vi "Untitled 1 (SubVI).vi"(11 "input string":string) -> ()   [LabVIEW 2017]
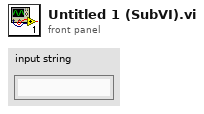
[diagram p1: front panel]
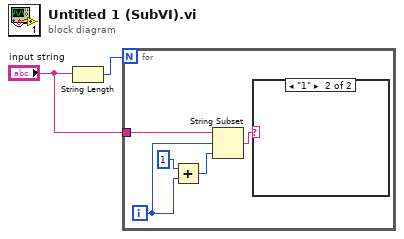
[diagram p0: block diagram]
diagram:
  n1 = String Length(string="input string") -> (length=w2:i32)
  n2 = for {
    N: w2 -> [_]
    tunnel: "input string" -> [w7]
    i -> [w4]
    n3 = Add(x=1, y=w4) -> (x+y=w5:i32)
    n4 = String Subset(string=w7, offset (0)=w4, length (rest)=w5) -> (substring=w3:string)
    n5 = case shown="\"1\"" w3 {
      frame "0", Default {
      }
      frame "1" {
      }
    }
  }
